vi "Write to lifter config_Running info.vi"(6 "error in (no error)":errorcluster, 9 "Insert Name":string) -> (0 "error out":errorcluster)   [LabVIEW 2019]
uses:
  <vilib>/Utility/config.llb/Write Key (String).vi
  <vilib>/Utility/config.llb/NI_LVConfig.lvlib
panel:
  out "appended path":path
  out "concatenated string":string
  in  "File Name":string="Lifter config"
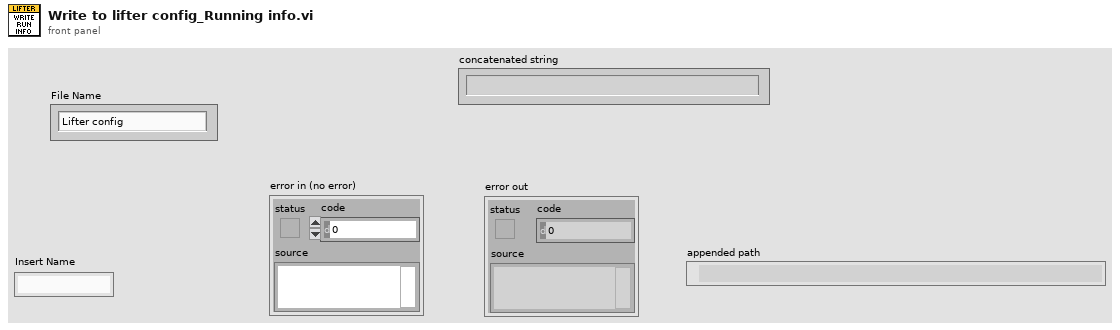
[diagram p1: front panel]
types:
  T1 = typedef "NI_LVConfig.lvlib/Config Data RefNum.ctl" = refnum<k1>
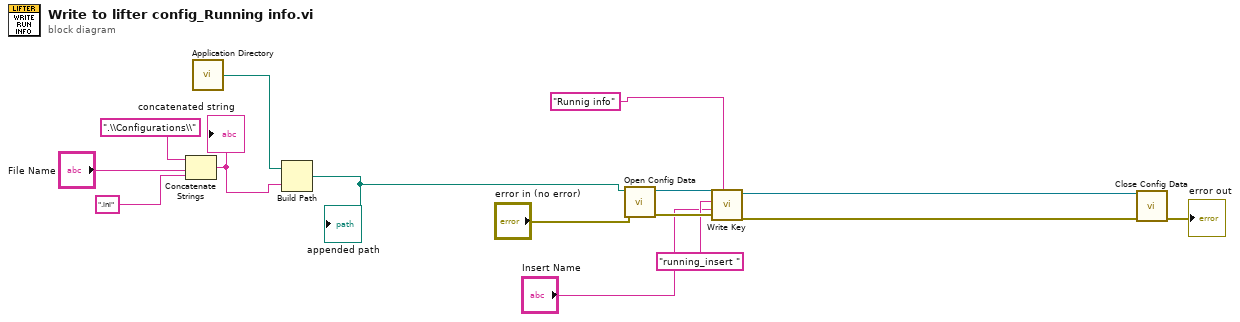
[diagram p0: block diagram]
diagram:
  n1 = Concatenate Strings(".\\Configurations\\" ("string"), "File Name", ".ini" ("string")) -> (w10:string)
  "concatenated string" <- w10
  n2 = call <vilib>:"Application Directory.vi"() -> ("Application Directory"=w8:path)
  n3 = Build Path(base path=w8, name or relative path=w10) -> (appended path=w5:path)
  "appended path" <- w5
  n4 = call <vilib>:"Open Config Data.vi"("error in (no error)"="error in (no error)", "configuration file path"=w5) -> ("error out"=w14:errorcluster, "refnum"=w15:T1)  [unwired: 7 in, 1 out]
  n5 = call-poly <vilib>:"Write Key.vi"("section"="Runnig info", "error in (no error)"=w14, "value"="Insert Name", "key"="running_insert ", "refnum"=w15) -> ("error out"=w2:errorcluster, "refnum out"=w1:T1)  [unwired: 4 in, 1 out]
  n6 = call <vilib>:"Close Config Data.vi"("error in (no error)"=w2, "refnum"=w1) -> ("error out"=→"error out":errorcluster)  [unwired: 8 in, 1 out]
